vi "dfd_Add Header to Filter String.vi"(9 "customer comments":string, 11 "string in":string) -> (3 "string out":string)   [LabVIEW 2017, in "NI_DigFilter_Process.lvlib"]
uses:
  <vilib>/addons/Digital Filter Design/NI_DigFilter_Process.lvlib
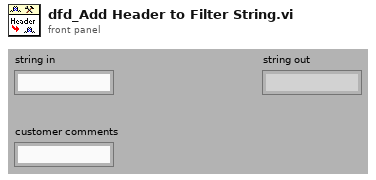
[diagram p1: front panel]
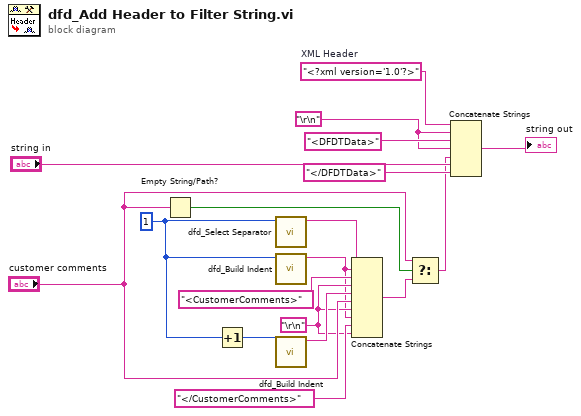
[diagram p0: block diagram]
diagram:
  w2 = "\r\n"
  w6 = 1 ("indent order")
  w16 = "\r\n"
  w15 = "<?xml version='1.0'?>"  # XML Header
  n1 = Empty String/Path?(string/path="customer comments") -> (empty?=w11:bool)
  n2 = Increment(x=w6) -> (x+1=w7:i32)
  n3 = call <vilib>:"dfd_Select Separator.vi"("indent order"=w6) -> ("separator"=w12:string)  [unwired: 10 out]
  n4 = call <vilib>:"dfd_Build Indent.vi"("indent order"=w6) -> ("tag indent"=w1:string)  [unwired: 10 out]
  n5 = call <vilib>:"dfd_Build Indent.vi"("indent order"=w7) -> ("tag indent"=w5:string)  [unwired: 10 out]
  n6 = Concatenate Strings(w12, w1, "<CustomerComments>" ("Substring"), w2, w5, "customer comments", w2, w1, "</CustomerComments>" ("Substring"), w2) -> (w9:string)
  n7 = Select(t="customer comments", s=w11, f=w9) -> (s? t:f=w10:string)
  n8 = Concatenate Strings(w15, w16, "<DFDTData>" ("Substring"), w16, w10, "string in", "</DFDTData>" ("Substring")) -> (→"string out":string)
